vi "SMBus Read Byte.vi"(6 "PEC":u8, 7 "SlaveAddr":u8, 8 "error in (no error)":errorcluster, 9 "SMBUSIndex":i32, 10 "DevIndex":i32, 11 "DevType":i32) -> (0 "error out":errorcluster, 2 "function return":i32, 3 "pData":string)   [LabVIEW 2012, in "ControlSMBus.lvlib"]
doc: "int WINAPI SMBus_ReadByte(int DevType,int DevIndex,int SMBUSIndex,unsigned char SlaveAddr,unsigned char *pData,unsigned char PEC);"
uses:
  ControlSMBus.lvlib
  Ginkgo_Driver.dll
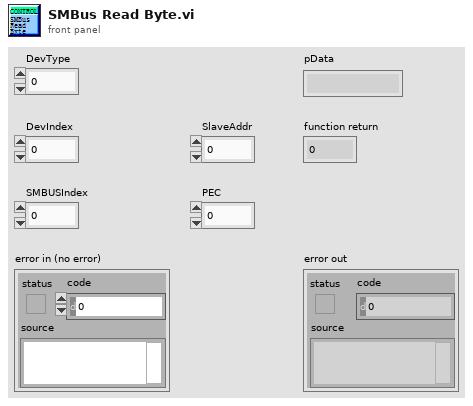
[diagram p1: front panel]
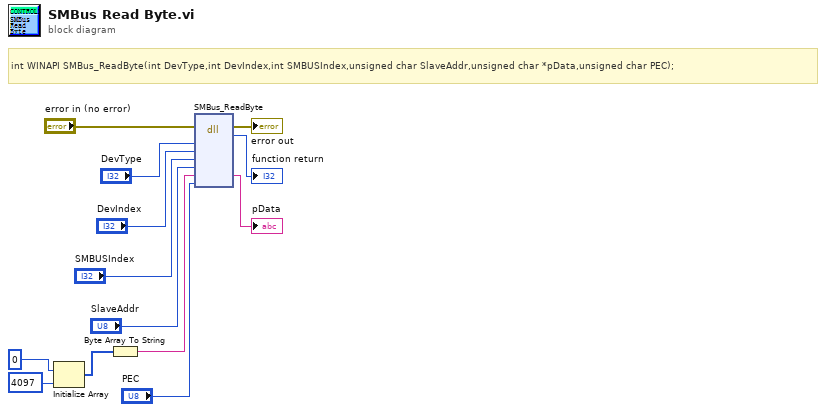
[diagram p0: block diagram]
diagram:
  # "int WINAPI SMBus_ReadByte(int DevType,int DevIndex,int SMBUSIndex,unsigned char SlaveAddr,unsigned char *pData,unsigned char PEC);"
  n1 = Initialize Array(u8 0 ("element"), 4097 ("dimension size")) -> (w8:u8[])
  n2 = Byte Array To String(unsigned byte array=w8) -> (string=w7:string)
  n3 = dll-call lib="E:/Project/vt_ginkgo/truck/Ginkgo Driver/vs2010/Ginkgo_USB-I2C_API_v2.0.3.0/lib/labview_64bit/ControlSMBus/Ginkgo_Driver.*" fn="SMBus_ReadByte"(error in="error in (no error)", "DevType"="DevType", "DevIndex"="DevIndex", "SMBUSIndex"="SMBUSIndex", "SlaveAddr"="SlaveAddr", "pData"=w7, "PEC"="PEC") -> (error out=→"error out":errorcluster, →"function return":i32, "pData"=→"pData":string)  [unwired: 7 in, 1 out]
